vi "chart series set trendline name lv.vi"(8 "error in (no error)":errorcluster, 10 "name":string, 11 "series":u32) -> (0 "error out":errorcluster)   [LabVIEW 8.6]
doc: "void chart_series_set_trendline_name_lv(lxw_chart_series series, const char *name);"
uses:
  pending_lvxlsxwriter/xlsxwriter.dll
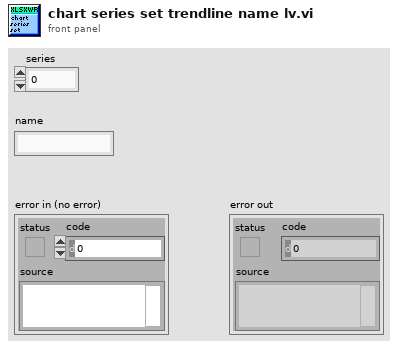
[diagram p1: front panel]
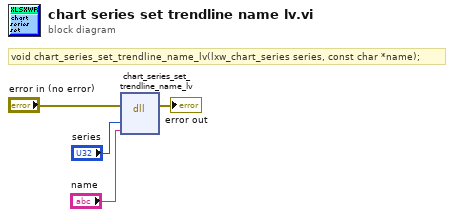
[diagram p0: block diagram]
diagram:
  # "void chart_series_set_trendline_name_lv(lxw_chart_series series, const char *name);"
  n1 = dll-call lib="C:/Users/WDAGUtilityAccount/Desktop/pending_lvxlsxwriter/xlsxwriter.*" fn="chart_series_set_trendline_name_lv"(error in="error in (no error)", "series"="series", "name"="name") -> (error out=→"error out":errorcluster)  [unwired: 5 in, 1 out]
